vi "Starter Kit 2.0 Custom FPGA Main.vi"() -> ()   [LabVIEW 2013]
doc: "This VI implements the low level control of the motors and sensor for the Starter Kit 2.0 robot. The functionality of this VI is similar to the fixed FPGA personality used by the Starter Kit API."
uses:
  <vilib>/Platform/TimedLoop/XDataNode/timing_clust.ctl
  <vilib>/Platform/TimedLoop/XDataNode/nitl_modes.ctl
  <vilib>/Platform/TimedLoop/XDataNode/wakeup.ctl
  <vilib>/robotics/Utilities/Encoder Count Encoding.ctl
  <vilib>/rvi/Emulation/niFpgaSctlEmulationGetInTimedLoop.vi
  <vilib>/rvi/Emulation/niFpgaProcessEmulError.vi
  <vilib>/rvi/Emulation/niFpgaEmulationReportErrorSimple.vi
  <vilib>/rvi/Emulation/niFpgaGetClockAttributes.vi
  <vilib>/rvi/Emulation/niFpgaCriticalErrorInLSC.vi
  <vilib>/robotics/Utilities/FPGA Utilities/Count Two Phase Digital Encoder.vi
  Support VIs/Starter Kit 2.0 FPGA Globals.vi
  <vilib>/robotics/Utilities/FPGA Utilities/Generate Digital Pulse (uSec).vi
  <vilib>/Platform/TimedLoop/XDataNode/XDataNode.xnode
  <vilib>/addons/control/pid/fpga.llb/XNode/niFpgaPID.xnode
  <vilib>/Platform/TimedLoop/XDataNode/XDNodeRunTimeDep.lvlib
  <vilib>/robotics/Utilities/NI_Robotics Utilities.lvlib
  <vilib>/robotics/Utilities/FPGA Utilities/NI_Robotics_FPGA Utilities.lvlib
  <instrlib>/Parallax PING)))/FPGA/NI_Robotics_Parallax PING))) (FPGA).lvlib
  <instrlib>/Hitec HS400 Series/FPGA/NI_Robotics_Hitec HS400 Series (FPGA).lvlib
panel:
  out "Right ccw count (pulses)":i32
  out "Left ccw count (pulses)":i32
  out "velocity (rad/s)":fxp<+/-,32,11> format="%.39g"
  out "Right Motos Ticks Count":i32
  out "Left Motor Ticks Count":i32
  out "Left Motor Pulse Width":u32
  out "Right Motor Pulse Width":u32
  in  "hs400_0_ccw offset":fxp<+/-,32,4>
  in  "hs400_0_ccw angle":fxp<+/-,32,4>
  out "PING)))_0_timeout":bool
  out "PING)))_0_dist":fxp<+,32,8> format="%.27g"
  out "DCmotor_1_ccw vel":fxp<+/-,32,11>
  out "DCmotor_0_ccw vel":fxp<+/-,32,11>
  in  "DCmotor_1_ccw vel sp":fxp<+/-,32,11>
  in  "DCmotor_0_ccw vel sp":fxp<+/-,32,11>
  in  "stop":bool
  in  "motor PID gains":T1={"proportional gain (Kc)"=0.25, "integral gain (Kc*Ts/Ti)"=0.08984375, "derivative gain (Kc*Td/Ts)"=0.01171875}
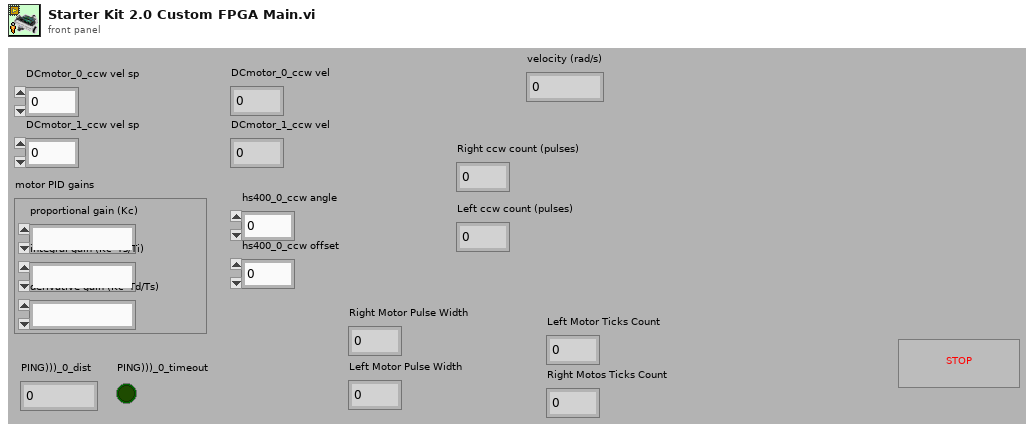
[diagram p1: front panel]
types:
  T1 = cluster{"proportional gain (Kc)":fxp<+/-,16,8>, "integral gain (Kc*Ts/Ti)":fxp<+/-,16,8>, "derivative gain (Kc*Td/Ts)":fxp<+/-,16,8>}
  T2 = cluster{"PID gains":cluster{"proportional gain (Kc)":fxp<+/-,16,8>, "integral gain (Kc*Ts/Ti)":fxp<+/-,16,8>, "derivative gain (Kc*Td/Ts)":fxp<+/-,16,8>}, "output range":cluster{"output high":fxp<+/-,16,16>, "output low":fxp<+/-,16,16>}, "setpoint":fxp<+/-,16,16>, "channel index":u16}
  T3 = cluster{"PID gains (x 2^8)":cluster{"proportional gain (Kc)":i16, "integral gain (Kc*Ts/Ti)":i16, "derivative gain (Kc*Td/Ts)":i16}, "output range":cluster{"output high":i16, "output low":i16}, "setpoint":i16, "channel index":u16}
  T4 = typedef "XDNodeRunTimeDep.lvlib/timing_clust.ctl" = cluster{"Expected End [f-1]":u64, "Actual End [f-1]":u64, "Finished Late? [f-1]":bool, "Expected End [i-1]":u64, "Actual End [i-1]":u64, "Finished Late? [i-1]":bool, "Expected Start [i]":u64, "Actual Start [i]":u64, "Expected Start [f]":u64, "Actual Start [f]":u64, "Source Name":string, "Structure Name":string, "Period":i64, "Deadline":i64, "Offset":i64, "Start":i64, "Priority":i32, "Timeout":i32, "Mode":T5, "Wakeup Reason":T6, "Error":errorcluster, "Source Type":string, "Secondary Source Type":string, "Global End Time":u64, "Global Start Time":u64, "Frame Duration":u64, "Iteration Duration":u64, "Assigned CPU":i32, "I/O Scan Engine Mode":u32}
  T5 = typedef "XDNodeRunTimeDep.lvlib/nitl_modes.ctl" = enum32{"No Change", "Process missed periods, maintain original phase", "Discard missed periods, maintain original phase", "Process missed periods, ignore original phase", "Discard missed periods, ignore original phase"}
  T6 = typedef "XDNodeRunTimeDep.lvlib/wakeup.ctl" = enum32{"Normal", "Aborted", "Asynchronous wakeup", "Timing source error", "Timed loop error", "Timeout"}
  T7 = typedef "NI_Robotics Utilities.lvlib/Encoder Count Encoding.ctl" = enum16{"X1", "X2", "X4"}
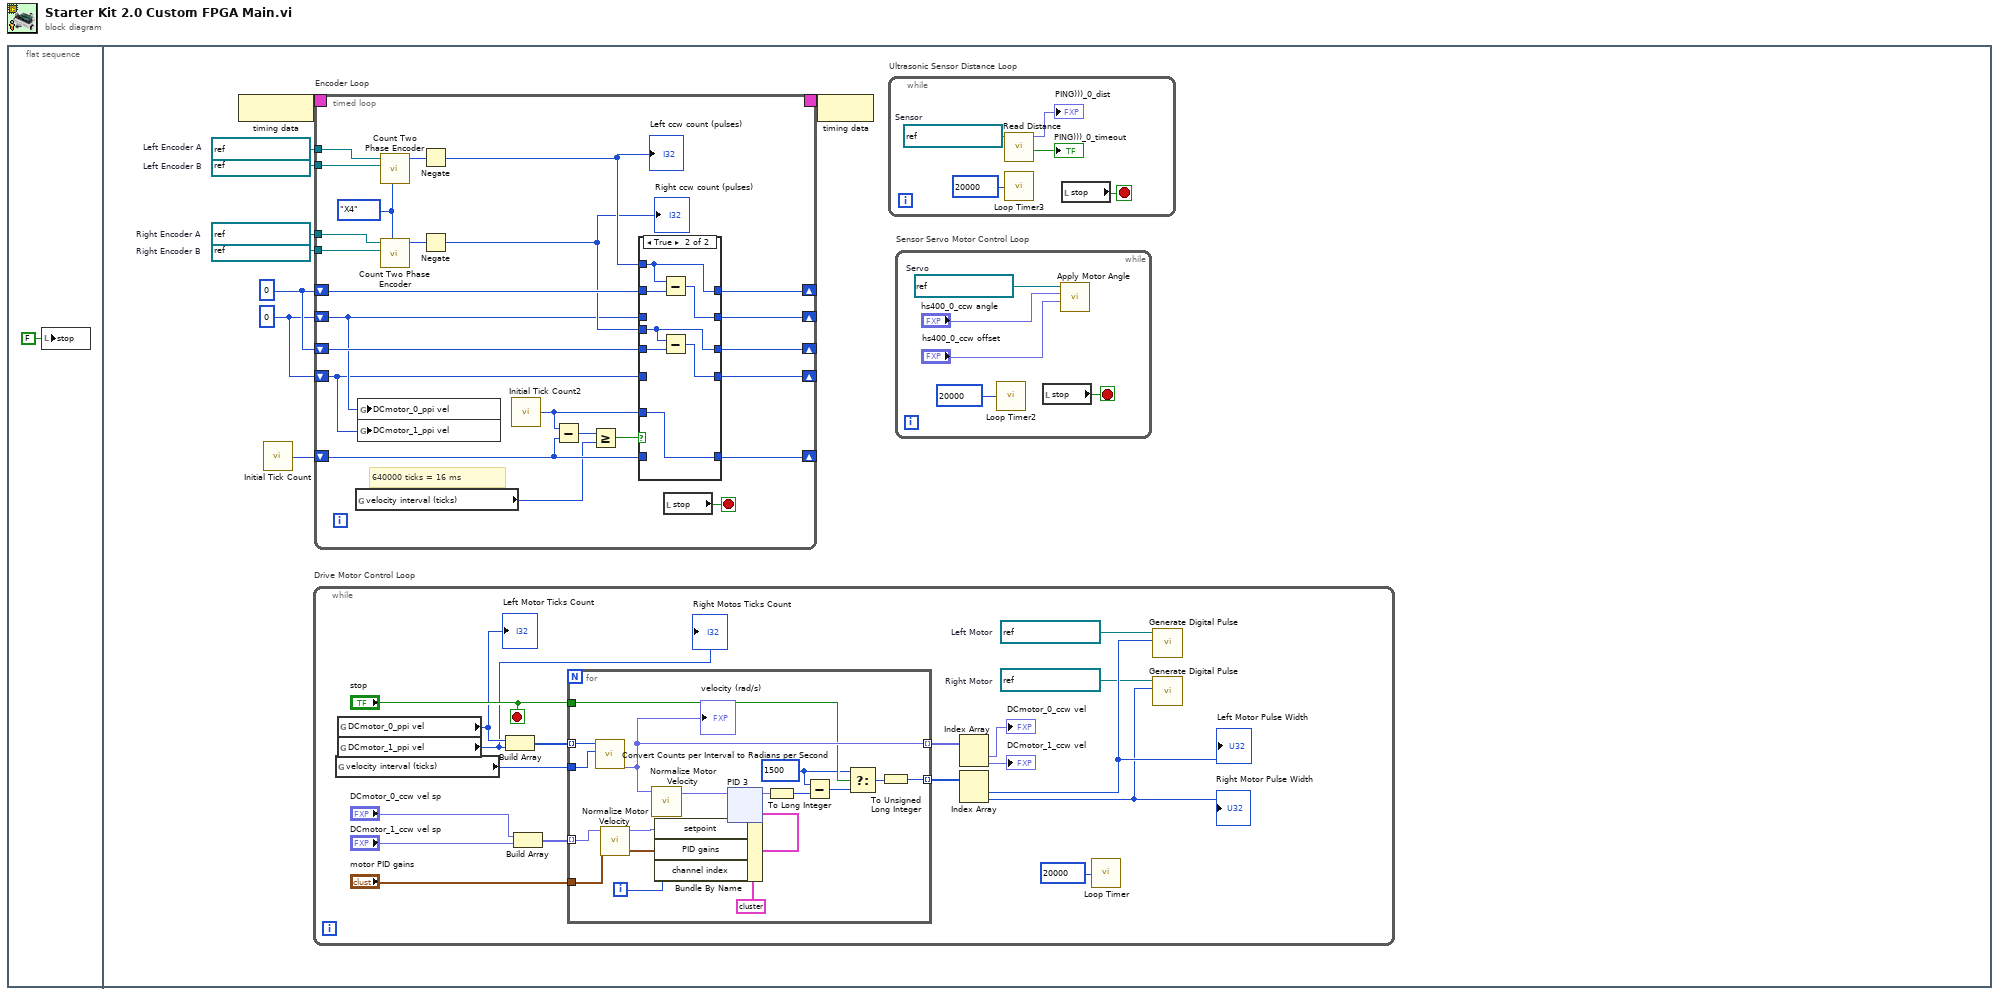
[diagram p0: block diagram]
diagram:
  n1 = flat-sequence {
    frame #0 {
      n2 = local write "stop"(FALSE ("stop")) -> ()
    }
    frame #1 {
      w2 = refnum<k21> "Port0/DIO3"  # Right Encoder B
      w3 = refnum<k21> "Port0/DIO2"  # Right Encoder A
      w4 = refnum<k21> "Port0/DIO1"  # Left Encoder B
      w5 = refnum<k21> "Port0/DIO0"  # Left Encoder A
      w6 = 0
      w7 = 0 ("Reset Position Value")
      n3 = node-c288() -> (w10:T4)
      n4 = call "Initial Tick Count"() -> ("Tick Count(Ticks)"=w8:u32)
      n5 = while "Drive Motor Control Loop" {
        stop <- "stop" stop-if-true
        w17 = refnum<k21> "Port0/DIO5"  # Right Motor
        w18 = refnum<k21> "Port0/DIO4"  # Left Motor
        n6 = global read "Starter Kit 2.0 FPGA Globals.vi" "velocity interval (ticks)"() -> (w13:u32)
        n7 = global read "Starter Kit 2.0 FPGA Globals.vi" "DCmotor_0_ppi vel"() -> (w12:i32)
        "Left Motor Ticks Count" <- w12
        n8 = global read "Starter Kit 2.0 FPGA Globals.vi" "DCmotor_1_ppi vel"() -> (w11:i32)
        "Right Motos Ticks Count" <- w11
        n9 = Build Array(w12, w11) -> (w26:i32[])
        n10 = Build Array("DCmotor_0_ccw vel sp", "DCmotor_1_ccw vel sp") -> (w24:fxp<+/-,32,11>[])
        n11 = for {
          tunnel: "motor PID gains" -> [w42]
          tunnel: w26 -> [w41] mode=indexing
          tunnel: w13 -> [w40]
          tunnel: [w39] -> w25 mode=indexing
          tunnel: w24 -> [w29] mode=indexing
          tunnel: "stop" -> [w33]
          tunnel: [w35] -> w23 mode=indexing
          i -> [w43]
          w32 = 1500 ("y")
          n12 = call "Convert Counts per Interval to Radians per Second.vi"("interval (ticks)"=w40, "velocity (pulses/interval)"=w41) -> ("velocity (rad/s)"=w39:fxp<+/-,32,11>)  [unwired: 9 in]
          "velocity (rad/s)" <- w39
          n13 = call "Normalize Motor Velocity.vi"("velocity (rad/s)"=w29) -> ("normalized velocity"=w36:fxp<+/-,16,16>)  [unwired: 10 in]
          n14 = call "Normalize Motor Velocity.vi"("velocity (rad/s)"=w39) -> ("normalized velocity"=w38:fxp<+/-,16,16>)  [unwired: 10 in]
          n15 = Bundle By Name(cluster=T2 {"PID gains"={"proportional gain (Kc)"=0.00390625, "integral gain (Kc*Ts/Ti)"=0.00390625, "derivative gain (Kc*Td/Ts)"=0.00390625}, "output range"={"output high"=500.0, "output low"=-500.0}, "setpoint"=0.0, "channel index"=0} ("configuration"), "setpoint"=w36, "PID gains"=w42, "channel index"=w43) -> (w44:T2)
          n16 = xnode ("PID 3")("process variable"=w38, "configuration"=w44) -> ("output"=w37:fxp<+/-,16,16>)  [unwired: 1 in, 1 out]
          n17 = To Long Integer(number=w37) -> (32bit integer=w34:i32)
          n18 = Subtract(x=w32, y=w34) -> (x-y=w31:i32)
          n19 = Select(t=w32, s=w33, f=w31) -> (s? t:f=w30:i32)
          n20 = To Unsigned Long Integer(number=w30) -> (unsigned 32bit integer=w35:u32)
        }
        n21 = Index Array(array=w25) -> (element #1=→"DCmotor_0_ccw vel":fxp<+/-,32,11>, element #2=→"DCmotor_1_ccw vel":fxp<+/-,32,11>)  [unwired: 2 in]
        n22 = Index Array(array=w23) -> (element #1=w22:u32, element #2=w19:u32)  [unwired: 2 in]
        "Right Motor Pulse Width" <- w19
        "Left Motor Pulse Width" <- w22
        n23 = call "Loop Timer"("Count(uSec)"=u32 20000) -> ()  [unwired: 1 out]
        n24 = call-poly <vilib>:"Generate Digital Pulse.vi"("pulse width (uSec)"=w22, "FPGA digital output"=w18) -> ()  [unwired: 10 in]
        n25 = call-poly <vilib>:"Generate Digital Pulse.vi"("pulse width (uSec)"=w19, "FPGA digital output"=w17) -> ()  [unwired: 10 in]
      }
      n26 = timed-loop "Encoder Loop" {
        timing: w10 -> [_]
        timing-out: [_] -> w9
        shift-right: [w99] -> _
        shift-left: w8 -> [w104]
        shift-right: [w100] -> _
        shift-left: w7 -> [w102]
        shift-right: [w101] -> _
        shift-left: w6 -> [w85]
        shift-right: [w97] -> _
        shift-left: w7 -> [w98]
        shift-right: [w96] -> _
        shift-left: w6 -> [w84]
        tunnel: w5 -> [w92]
        tunnel: w4 -> [w91]
        tunnel: w3 -> [w89]
        tunnel: w2 -> [w88]
        stop <- w93 stop-if-true
        w86 = Encoder_Count_Encoding."X4" ("count multiplier (X1)")
        # "640000 ticks = 16 ms"
        n27 = global read "Starter Kit 2.0 FPGA Globals.vi" "velocity interval (ticks)"() -> (w83:u32)
        n28 = global write "Starter Kit 2.0 FPGA Globals.vi" "DCmotor_0_ppi vel"(w85) -> ()
        n29 = global write "Starter Kit 2.0 FPGA Globals.vi" "DCmotor_1_ppi vel"(w84) -> ()
        n30 = call-poly <vilib>:"Count Two Phase Encoder.vi"("count encoding (X1)"=w86, "phase B FPGA digital input"=w91, "phase A FPGA digital input"=w92) -> ("new count"=w90:i32)  [unwired: 7 in, 1 out]
        n31 = call-poly <vilib>:"Count Two Phase Encoder.vi"("count encoding (X1)"=w86, "phase B FPGA digital input"=w88, "phase A FPGA digital input"=w89) -> ("new count"=w87:i32)  [unwired: 7 in, 1 out]
        n32 = Negate(x=w90) -> (-x=w95:i32)
        "Left ccw count (pulses)" <- w95
        n33 = Negate(x=w87) -> (-x=w94:i32)
        "Right ccw count (pulses)" <- w94
        n34 = call "Initial Tick Count2"() -> ("Tick Count(Ticks)"=w103:u32)
        n35 = Subtract(x=w103, y=w104) -> (x-y=w106:u32)
        n36 = Greater Or Equal?(x=w106, y=w83) -> (x >= y?=w105:bool)
        n37 = case shown="True" w105 {
          tunnel: w103 -> [_ w117]
          tunnel: w104 -> [w111 _]
          tunnel: [w111 w117] -> w99
          tunnel: w102 -> [w110 w118]
          tunnel: [w110 w116] -> w100
          tunnel: w95 -> [_ w116]
          tunnel: [w109 w115] -> w101
          tunnel: w85 -> [w109 _]
          tunnel: w98 -> [w108 w114]
          tunnel: w84 -> [w107 _]
          tunnel: [w108 w113] -> w97
          tunnel: [w107 w112] -> w96
          tunnel: w94 -> [_ w113]
          frame False {
          }
          frame True {
            n38 = Subtract(x=w116, y=w118) -> (x-y=w115:i32)
            n39 = Subtract(x=w113, y=w114) -> (x-y=w112:i32)
          }
        }
        n40 = local read "stop"() -> (w93:bool)
      }
      n41 = node-c288(w9) -> ()
      n42 = while "Ultrasonic Sensor Distance Loop" {
        stop <- w81 stop-if-true
        w78 = refnum<k21> "Port0/DIO6"  # Sensor
        n43 = call <instrlib>:"Read Distance.vi"("trigger/echo line"=w78) -> ("timed out?"=→"PING)))_0_timeout":bool, "distance (m)"=→"PING)))_0_dist":fxp<+,32,8>)  [unwired: 9 in]
        n44 = call "Loop Timer3"("Count(uSec)"=u32 20000 ("sensor period (15000 us)")) -> ()  [unwired: 1 out]
        n45 = local read "stop"() -> (w81:bool)
      }
      n46 = while "Sensor Servo Motor Control Loop" {
        stop <- w77 stop-if-true
        w76 = refnum<k21> "Port0/DIO7"  # Servo
        n47 = call "Loop Timer2"("Count(uSec)"=u32 20000) -> ()  [unwired: 1 out]
        n48 = local read "stop"() -> (w77:bool)
        n49 = call <instrlib>:"Apply Motor Angle.vi"("ccw angle offset (rad)"="hs400_0_ccw offset", "ccw angle (rad)"="hs400_0_ccw angle", "digital output line"=w76) -> ()  [unwired: 9 in]
      }
    }
  }
